vi "未命名 5.vi"() -> ()   [LabVIEW 2012]
panel:
  out "强度图":i32[][](graph)
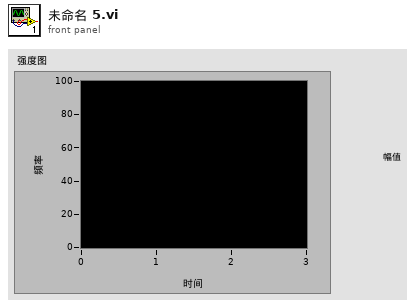
[diagram p1: front panel]
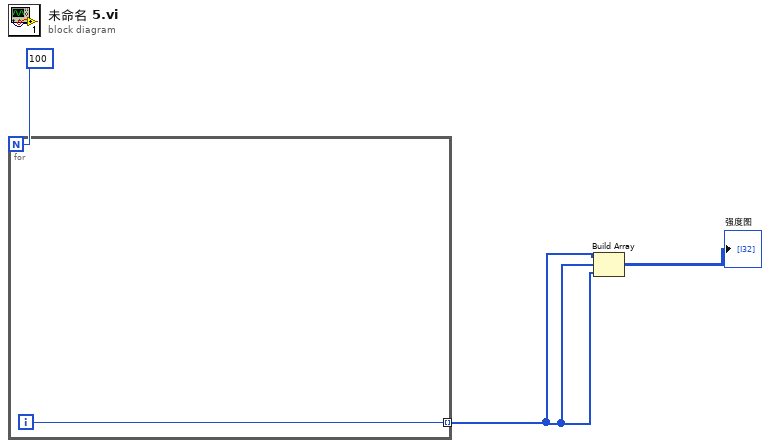
[diagram p0: block diagram]
diagram:
  n1 = for {
    N: 100 -> [_]
    tunnel: [w4] -> w1 mode=indexing
    i -> [w4]
  }
  n2 = Build Array(w1, w1, w1) -> (→"强度图":i32[][])
